vi "PH_Calorimeter_USB.Calc Integration Time.vi"(2 "Data without Offset":sgl[](array[numeric]) format="%.2f", 3 "Time scale [s]":dbl[](array[numeric]) format="%.2f") -> (4 "Integration Time [s]":dbl format="%.2f")   [LabVIEW 2014, in "PH_Calorimeter_USB.lvlib"]
doc: "This VI calculates the integration time. It searches for the maximum of \"data in\" and gives out the time from the related \"time in\" array."
uses:
  PH_Calorimeter_USB.lvlib
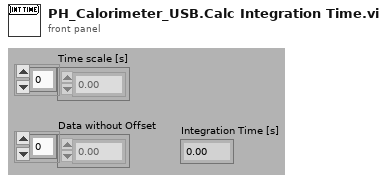
[diagram p1: front panel]
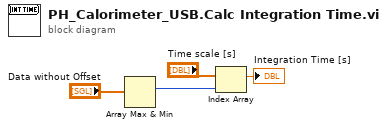
[diagram p0: block diagram]
diagram:
  n1 = Array Max & Min(array="Data without Offset") -> (max index (indices)=w1:i32)  [unwired: 3 out]
  n2 = Index Array(array="Time scale [s]", index=w1) -> (element=→"Integration Time [s]":dbl)
